vi "insert channel.vi"(8 "number of available channels":u16, 9 "Volts":T1={"conversion matrix"=[[0.0, 0.0], [0.0, 0.0], [0.0, 0.0], [0.0, 0.0], [0.0, 0.0], [0.0, 0.0]], "units"="volts", "name"="", "scale type"=enum."Volts", "offset (volts)"=0.0, "second channel"=0, "correspondence table"=[], "offset (physical units)"=0.0, "pH scale"={"Buffers"=[], "Temperature"=0.0}, "D.O."={"Temperature"=0.0, "K"=0.0, "barometric pressure"=0.0}, "Photometer data"={"Dark Voltage"=0.0, "Blank Voltage"=0.0, "Standards"=[]}} {"D.O."."K" format="%.6f"; "D.O."."Temperature" format="%.2f"; "pH scale"."Buffers"."V/T" format="%.5f"; "pH scale"."Buffers"."Buffer" format="%.2f"; "pH scale"."Temperature" format="%.2f"; "offset (physical units)" format="%.5f"; "correspondence table"."volts" format="%.4f"; "correspondence table"."physical units" format="%.4f"; "second channel" min=-1; "offset (volts)" format="%.5f"; "conversion matrix" format="%.4e"}, 11 "Index":u32) -> (2 "Sensor Array out":T7, 3 "Index out":u32)   [LabVIEW 2015]
uses:
  DAQ configuration/Sensor array.ctl
  DAQ configuration/channel identifier.ctl
  conversion.ctl
  DAQ configuration/scale type.ctl
  correspondence table.ctl
  pH/pH scale.ctl
  Dissolved Oxygen/DO scale.ctl
  Spectrophotometer/Photometer calibration data.ctl
  DAQ configuration/Sensor buffer command.ctl
panel:
  # "C"
  # "kPa"
  # "C"
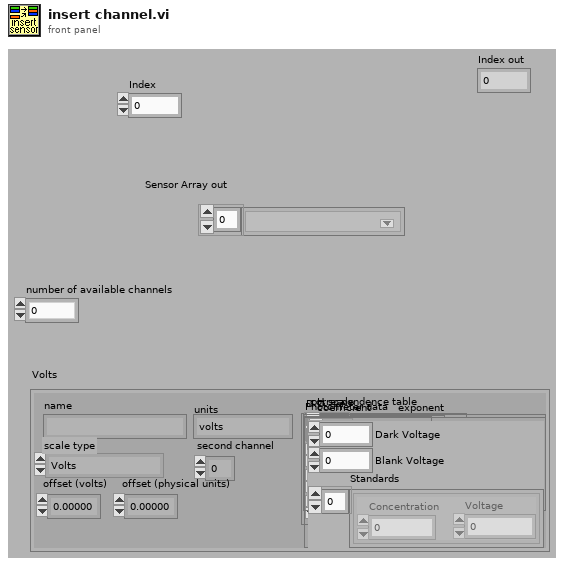
[diagram p1: front panel]
types:
  T1 = typedef "conversion.ctl" = cluster{"conversion matrix":sgl[][], "units":string, "name":string, "scale type":T2, "offset (volts)":dbl, "second channel":i8, "correspondence table":T3, "offset (physical units)":dbl, "pH scale":T4, "D.O.":T5, "Photometer data":T6}
  T2 = typedef "scale type.ctl" = enum16{"Volts", "Polynomial", "Correspondence Table", "pH", "Dissolved Oxygen", "Quadratic", "Photometer"}
  T3 = typedef "correspondence table.ctl" = cluster{"physical units":dbl, "volts":dbl}[]
  T4 = typedef "pH scale.ctl" = cluster{"Buffers":cluster{"Buffer":dbl, "Calibrated":bool, "V/T":dbl}[], "Temperature":dbl}
  T5 = typedef "DO scale.ctl" = cluster{"Temperature":dbl, "K":dbl, "barometric pressure":dbl}
  T6 = typedef "Photometer calibration data.ctl" = cluster{"Dark Voltage":dbl, "Blank Voltage":dbl, "Standards":cluster{"Concentration":dbl, "Voltage":dbl}[]}
  T7 = typedef "Sensor array.ctl" = T8[]
  T8 = typedef "channel identifier.ctl" = u16
  T9 = typedef "Sensor buffer command.ctl" = enum16{"read average", "read recent", "read all", "write", "set buffer size", "Read channel config", "Write channel config", "clear"}
  T10 = typedef "Channel config.ctl" = cluster{"Channel Indices":T8[], "AI Max voltage":dbl[], "Calibration matrix":T11}
  T11 = typedef "calib array.ctl" = T1[]
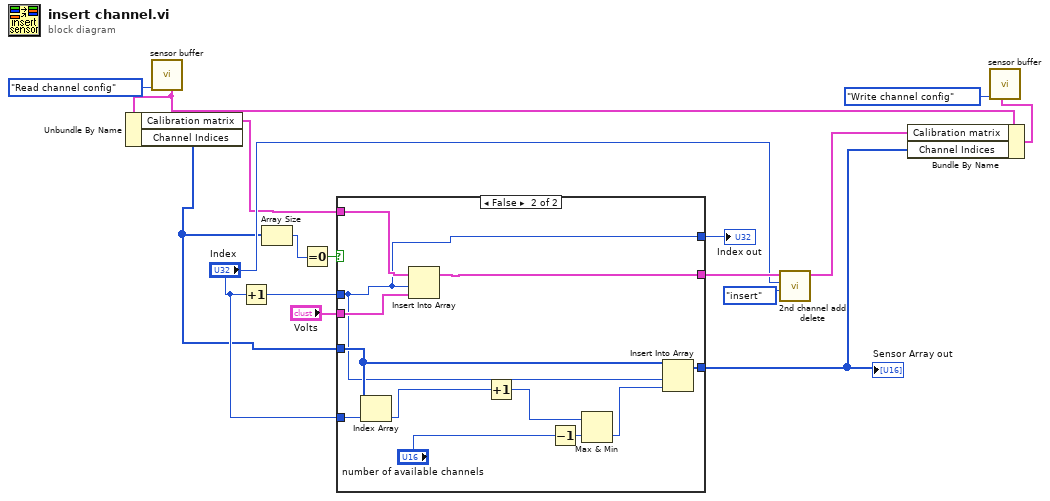
[diagram p0: block diagram]
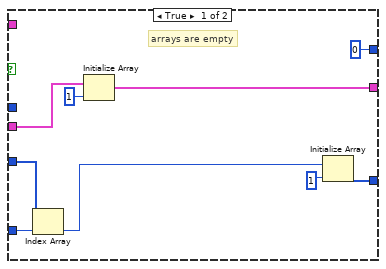
[diagram p2: hidden frame]
diagram:
  n1 = call "sensor buffer.vi"("command"=Sensor_buffer_command."Read channel config") -> ("Channel Config out"=w6:T10)  [unwired: 6 in, 4 out]
  n2 = Unbundle By Name(w6) -> ("Calibration matrix"=w5:T11, "Channel Indices"=w4:T8[])
  n3 = Increment(x="Index") -> (x+1=w16:u32)
  n4 = Array Size(array=w4) -> (size(s)=w15:i32)
  n5 = Equal To 0?(x=w15) -> (x = 0?=w14:bool)
  n6 = case shown="False" w14 {
    tunnel: "Index" -> [w25 w37]
    tunnel: w16 -> [_ w31]
    tunnel: w5 -> [_ w36]
    tunnel: w4 -> [w20 w35]
    tunnel: [w19 w34] -> w2
    tunnel: [w23 w33] -> w11
    tunnel: "Volts" -> [w24 w32]
    tunnel: [u32 0 ("Index out") w31] -> w12
    frame True {
      # "arrays are empty"
      n7 = Index Array(array=w20, index=w25) -> (element=w17:T8)
      n8 = Initialize Array(w24, 1 ("Dimension Size")) -> (w23:T1[])
      n9 = Initialize Array(w17, 1 ("Dimension Size")) -> (w19:T8[])
    }
    frame False {
      n10 = Index Array(array=w35, index=w37) -> (element=w30:T8)
      n11 = Insert Into Array(array=w36, index=w31, new element=w32) -> (w33:T11)
      n12 = Increment(x=w30) -> (x+1=w28:T8)
      n13 = Decrement(x="number of available channels") -> (x-1=w26:u16)
      n14 = Max & Min(x=w28, y=w26) -> (min(x,y)=w27:T8)  [unwired: 1 out]
      n15 = Insert Into Array(array=w35, index=w31, new element=w27) -> (w34:T8[])
    }
  }
  "Sensor Array out" <- w2
  "Index out" <- w12
  n16 = call "2nd channel add delete.vi"("action"=enum16{"delete", "insert"}."insert", "Index"="Index", "Calibration array"=w11) -> ("Calibration array out"=w3:T11)  [unwired: 8 in]
  n17 = Bundle By Name(cluster=w6, "Calibration matrix"=w3, "Channel Indices"=w2) -> (w1:T10)
  n18 = call "sensor buffer.vi"("Channel Config"=w1, "command"=Sensor_buffer_command."Write channel config") -> ()  [unwired: 5 in, 5 out]
